vi "Variant to string.vi"(8 "error in (no error)":errorcluster, 11 "Variant":variant) -> (0 "error out":errorcluster, 3 "String":string)   [LabVIEW 2020, in "LUnit Test Case.lvclass"]
uses:
  LUnit Test Case.lvclass
  <vilib>/Utility/Data Type/NI_Data Type.lvlib
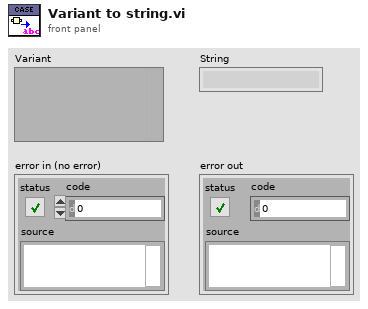
[diagram p1: front panel]
types:
  T1 = typedef "NI_Data Type.lvlib/Data Type.ctl" = enum8{"Invalid Type", "Void", "I8", "I16", "I32", "I64", "U8", "U16", "U32", "U64", "Single Float", "Double Float", "Extended Float", "Single Complex", "Double Complex", "Extended Complex", "Enum U8", "Enum U16", "Enum U32", "Enum U64", "Single Float With Unit", "Double Float With Unit", "Extended Float With Unit", "Single Complex with Unit", "Double Complex with Unit", "Extended Complex with Unit", "Boolean", "String", "Path", "Picture", "Tag", "Array", "Cluster", "Variant", "LV Variant", "Waveform", "Timestamp", "Digital Waveform", "Digital Data", "ExpressData", "Refnum", "External Data", "VI", "Poly VI", "LabVIEW Class Instance", "Fixed Point", "Set Collection", "Map Collection"}
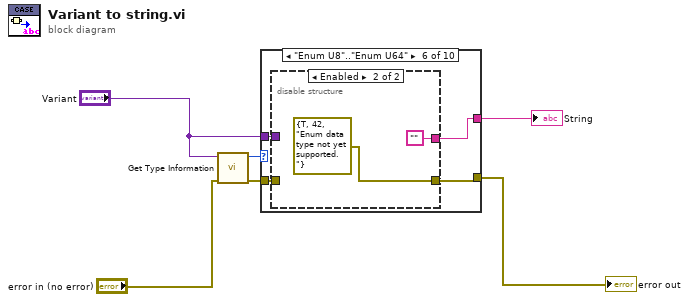
[diagram p0: block diagram]
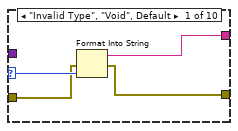
[diagram p2: hidden frame]
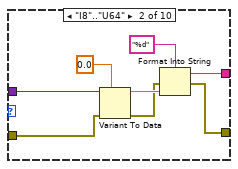
[diagram p3: hidden frame]
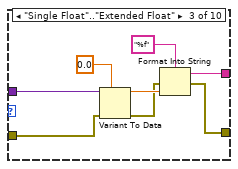
[diagram p4: hidden frame]
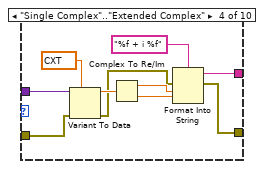
[diagram p5: hidden frame]
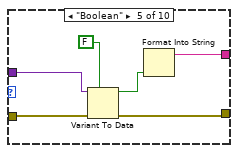
[diagram p6: hidden frame]
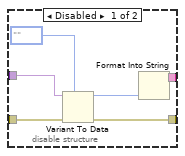
[diagram p7: hidden frame]
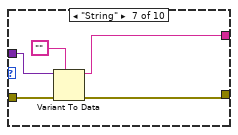
[diagram p8: hidden frame]
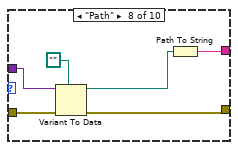
[diagram p9: hidden frame]
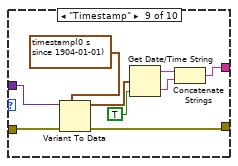
[diagram p10: hidden frame]
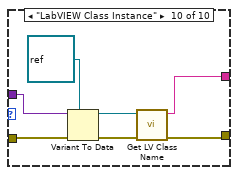
[diagram p11: hidden frame]
diagram:
  n1 = call <vilib>:"Get Type Information.vi"("error in (no error)"="error in (no error)", "variant"="Variant") -> ("error out"=w4:errorcluster, "type"=w5:T1)  [unwired: 5 in, 3 out]
  n2 = case shown="\"Enum U8\"..\"Enum U64\"" w5 {
    selector: w5 -> [w10 _ _ _ _ _ _ _ _ _]
    tunnel: "Variant" -> [_ w18 w26 w36 w41 w46 w58 w64 w73 w81]
    tunnel: [w7 w14 w22 w34 w38 w43 w56 w62 w68 w75] -> w6
    tunnel: w4 -> [w9 w12 w20 w33 w42 w45 w59 w65 w74 w79]
    tunnel: [w8 w11 w19 w32 w37 w44 w55 w60 w67 w76] -> w3
    frame "Invalid Type", "Void", Default {
      n3 = Format Into String(error in=w9, w10) -> (resulting string=w7:string, error out=w8:errorcluster)  [unwired: 2 in]
    }
    frame "I8".."U64" {
      n4 = Variant To Data(error in=w12, type=0.0 ("double precision float"), Variant=w18) -> (data=w16:dbl, error out=w13:errorcluster)
      n5 = Format Into String(format string="%d", error in=w13, w16) -> (resulting string=w14:string, error out=w11:errorcluster)  [unwired: 1 in]
    }
    frame "Single Float".."Extended Float" {
      n6 = Variant To Data(error in=w20, type=0.0 ("double precision float"), Variant=w26) -> (data=w24:dbl, error out=w21:errorcluster)
      n7 = Format Into String(format string="%f", error in=w21, w24) -> (resulting string=w22:string, error out=w19:errorcluster)  [unwired: 1 in]
    }
    frame "Single Complex".."Extended Complex" {
      n8 = Variant To Data(error in=w33, type=cxt 0.0+0.0i, Variant=w36) -> (data=w30:cxt, error out=w27:errorcluster)
      n9 = Complex To Re/Im(x + iy=w30) -> (x=w29:ext, y=w28:ext)
      n10 = Format Into String(format string="%f + i %f", error in=w27, w29, w28) -> (resulting string=w34:string, error out=w32:errorcluster)  [unwired: 1 in]
    }
    frame "Boolean" {
      n11 = Variant To Data(error in=w42, type=FALSE, Variant=w41) -> (data=w39:bool, error out=w37:errorcluster)
      n12 = Format Into String(w39) -> (resulting string=w38:string)  [unwired: 3 in, 1 out]
    }
    frame "Enum U8".."Enum U64" {
      n13 = disable-structure shown="Enabled" {
        disable-tunnel: w46 -> [w52 _]
        disable-tunnel: w45 -> [w50 _]
        disable-tunnel: [w49 errorcluster {"status"=TRUE, "code"=42, "source"="Enum data type not yet supported. "} ("error out")] -> w44
        disable-tunnel: [w47 ""] -> w43
        frame Disabled {
          n14 = Variant To Data(error in=w50, type=enum16{""}."", Variant=w52) -> (data=w48:enum16{""}, error out=w49:errorcluster)
          n15 = Format Into String(w48) -> (resulting string=w47:string)  [unwired: 3 in, 1 out]
        }
        frame Enabled {
        }
      }
    }
    frame "String" {
      n16 = Variant To Data(error in=w59, type="", Variant=w58) -> (data=w56:string, error out=w55:errorcluster)
    }
    frame "Path" {
      n17 = Variant To Data(error in=w65, type=path "", Variant=w64) -> (data=w61:path, error out=w60:errorcluster)
      n18 = Path To String(path=w61) -> (string=w62:string)
    }
    frame "Timestamp" {
      n19 = Variant To Data(error in=w74, type=timestamp(0 s since 1904-01-01), Variant=w73) -> (data=w71:timestamp, error out=w67:errorcluster)
      n20 = Get Date/Time String(seconds (now)=w71, want seconds? (F)=TRUE) -> (date string=w70:string, time string=w69:string)  [unwired: 1 in]
      n21 = Concatenate Strings(w70, w69) -> (w68:string)
    }
    frame "LabVIEW Class Instance" {
      n22 = Variant To Data(error in=w79, type=refnum<class> refnum ("object"), Variant=w81) -> (data=w78:refnum<class>, error out=w77:errorcluster)
      n23 = call <vilib>:"Get LV Class Name.vi"("error in (no error)"=w77, "object"=w78) -> ("error out"=w76:errorcluster, "class name"=w75:string)  [unwired: 8 in]
    }
  }
  "error out" <- w3
  "String" <- w6
